vi "String - Ctl to String.vi"(11 "reference":refnum<vi>) -> (1 "String":string, 2 "Label.Text":string, 3 "reference out":refnum<vi>)   [LabVIEW 2013]
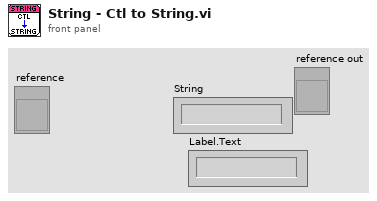
[diagram p1: front panel]
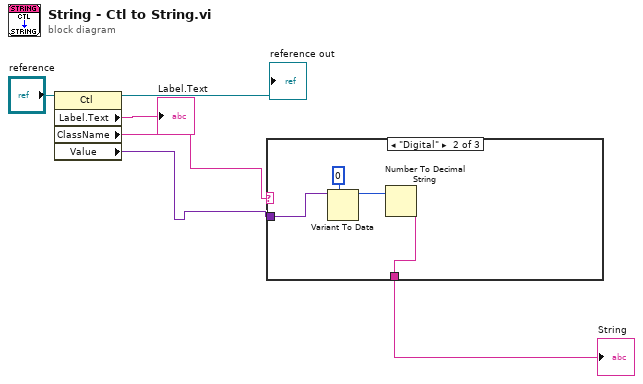
[diagram p0: block diagram]
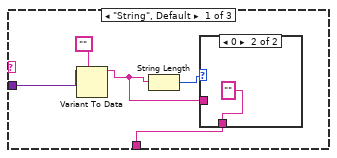
[diagram p2: hidden frame]
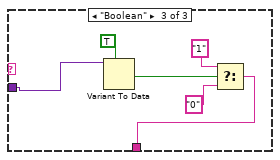
[diagram p4: hidden frame]
diagram:
  n1 = property class="Ctl"(reference="reference") -> (reference out=→"reference out":refnum<vi>, "Label.Text"=→"Label.Text":string, "ClassName"=w3:string, "Value"=w5:variant)  [unwired: 1 in, 1 out]
  n2 = case shown="\"Digital\"" w3 {
    tunnel: w5 -> [w11 w17 w23]
    tunnel: [w7 w14 w18] -> w6
    frame "String", Default {
      n3 = Variant To Data(type="", Variant=w11) -> (data=w8:string)  [unwired: 1 in, 1 out]
      n4 = String Length(string=w8) -> (length=w9:i32)
      n5 = case shown="0" w9 {
        tunnel: w8 -> [w12 _]
        tunnel: [w12 ""] -> w7
        frame 1, Default {
        }
        frame 0 {
        }
      }
    }
    frame "Digital" {
      n6 = Variant To Data(type=0, Variant=w17) -> (data=w15:i32)  [unwired: 1 in, 1 out]
      n7 = Number To Decimal String(number=w15) -> (decimal integer string=w14:string)  [unwired: 1 in]
    }
    frame "Boolean" {
      n8 = Variant To Data(type=TRUE, Variant=w23) -> (data=w21:bool)  [unwired: 1 in, 1 out]
      n9 = Select(t="1", s=w21, f="0") -> (s? t:f=w18:string)
    }
  }
  "String" <- w6
